vi "BRig_RT_comm_webdav_upload__gatherFilenames.vi"() -> (2 "output_arrBlank":bool[](array[boolean]), 3 "output_arrFilenames":string[](array[string]), 5 "output_n":i32)   [LabVIEW 2014]
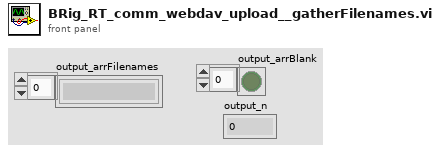
[diagram p1: front panel]
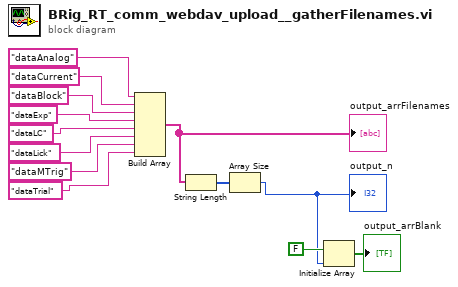
[diagram p0: block diagram]
diagram:
  n1 = Build Array("dataAnalog" ("input_filename"), "dataCurrent" ("input_filename"), "dataBlock" ("input_filename"), "dataExp" ("input_filename"), "dataLC" ("input_filename"), "dataLick" ("input_filename"), "dataMTrig" ("input_filename"), "dataTrial" ("input_filename")) -> (w3:string[])
  "output_arrFilenames" <- w3
  n2 = String Length(string=w3) -> (length=w2:i32[])
  n3 = Array Size(array=w2) -> (size(s)=w1:i32)
  "output_n" <- w1
  n4 = Initialize Array(FALSE, w1) -> (→"output_arrBlank":bool[])
